vi "Split.vi"(8 "error in (no error)":errorcluster, 11 "SnailNum in":refnum<class "SnailNum.lvclass">) -> (0 "error out":errorcluster, 2 "Did Split?":bool, 3 "SnailNum out":refnum<class "SnailNum.lvclass">)   [LabVIEW 2020, in "SnailNum.lvclass"]
uses:
  SnailNum.lvclass
  SnailNum.lvclass/SnailNum.ctl
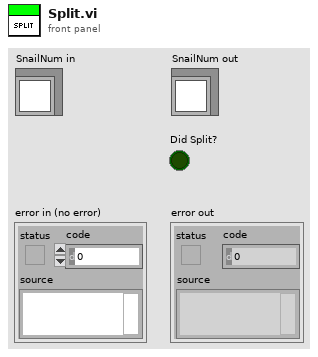
[diagram p1: front panel]
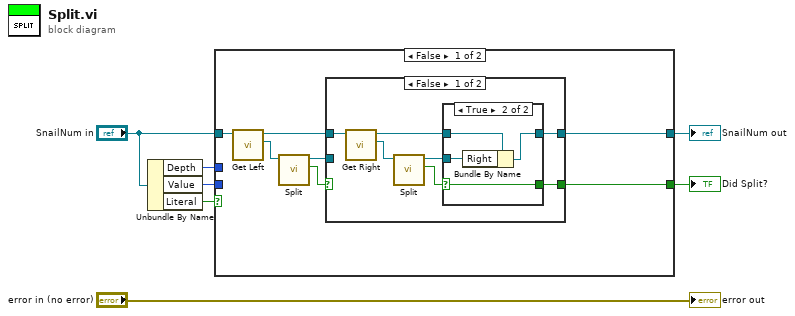
[diagram p0: block diagram]
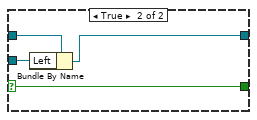
[diagram p3: hidden frame]
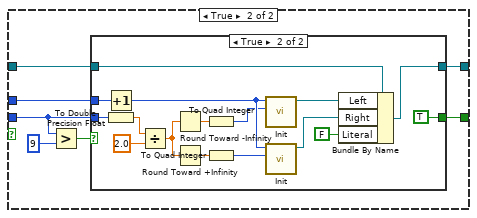
[diagram p4: hidden frame]
diagram:
  n1 = Unbundle By Name("SnailNum in") -> ("Depth"=w2:i32, "Value"=w3:i64, "Literal"=w4:bool)
  n2 = case shown="False" w4 {
    tunnel: [w10 w32] -> w6
    tunnel: "SnailNum in" -> [w9 w34]
    tunnel: w3 -> [_ w35]
    tunnel: w2 -> [_ w33]
    tunnel: [w8 w31] -> w1
    frame False {
      n3 = call "Get Left.vi"("SnailNum in"=w9) -> ("Left"=w14:refnum<class "SnailNum.lvclass">, "SnailNum out"=w13:refnum<class "SnailNum.lvclass">)  [unwired: 8 in, 1 out]
      n4 = call "Split.vi"("SnailNum in"=w14) -> ("Did Split?"=w12:bool, "SnailNum out"=w11:refnum<class "SnailNum.lvclass">)  [unwired: 8 in, 1 out]
      n5 = case shown="False" w12 {
        selector: w12 -> [_ w27]
        tunnel: w13 -> [w21 w30]
        tunnel: w11 -> [_ w29]
        tunnel: [w16 w28] -> w10
        tunnel: [w15 w27] -> w8
        frame False {
          n6 = call "Get Right.vi"("SnailNum in"=w21) -> ("Right"=w20:refnum<class "SnailNum.lvclass">, "SnailNum out"=w17:refnum<class "SnailNum.lvclass">)  [unwired: 8 in, 1 out]
          n7 = call "Split.vi"("SnailNum in"=w20) -> ("Did Split?"=w19:bool, "SnailNum out"=w18:refnum<class "SnailNum.lvclass">)  [unwired: 8 in, 1 out]
          n8 = case shown="True" w19 {
            selector: w19 -> [_ w23]
            tunnel: w18 -> [_ w25]
            tunnel: w17 -> [w22 w26]
            tunnel: [w22 w24] -> w16
            tunnel: [_ w23] -> w15
            frame False {
            }
            frame True {
              n9 = Bundle By Name(cluster=w26, "Right"=w25) -> (w24:refnum<class "SnailNum.lvclass">)
            }
          }
        }
        frame True {
          n10 = Bundle By Name(cluster=w30, "Left"=w29) -> (w28:refnum<class "SnailNum.lvclass">)
        }
      }
    }
    frame True {
      n11 = Greater?(x=w35, y=i64 9) -> (0:w36:bool)
      n12 = case shown="True" w36 {
        tunnel: w35 -> [_ w52]
        tunnel: w34 -> [w38 w44]
        tunnel: w33 -> [_ w54]
        tunnel: [w38 w40] -> w32
        tunnel: [_ TRUE] -> w31
        frame False {
        }
        frame True {
          n13 = Increment(x=w54) -> (x+1=w53:i32)
          n14 = To Double Precision Float(number=w52) -> (double precision float=w51:dbl)
          n15 = Divide(x=w51, y=2.0) -> (x/y=w46:dbl)
          n16 = Round Toward -Infinity(1:w46) -> (0:w49:dbl)
          n17 = Round Toward +Infinity(x=w46) -> (ceil(x): smallest int >= x=w47:dbl)
          n18 = To Quad Integer(1:w49) -> (0:w48:i64)
          n19 = To Quad Integer(1:w47) -> (0:w45:i64)
          n20 = call "Init.vi"("Value"=w48, "Depth"=w53) -> ("SnailNum out"=w43:refnum<class "SnailNum.lvclass">)  [unwired: 8 in, 1 out]
          n21 = call "Init.vi"("Value"=w45, "Depth"=w53) -> ("SnailNum out"=w42:refnum<class "SnailNum.lvclass">)  [unwired: 8 in, 1 out]
          n22 = Bundle By Name(cluster=w44, "Left"=w43, "Right"=w42, "Literal"=FALSE) -> (w40:refnum<class "SnailNum.lvclass">)
        }
      }
    }
  }
  "SnailNum out" <- w6
  "Did Split?" <- w1
  "error out" <- "error in (no error)"
